vi "写入数据.vi"(8 "error in (no error)":errorcluster caption="错误输入（无错误）", 10 "数据":dbl[](array[numeric]), 11 "DAQ输入":refnum<class "DAQ.lvclass">) -> (0 "error out":errorcluster caption="错误输出", 3 "DAQ输出":refnum<class "DAQ.lvclass">)   [LabVIEW 2015]
uses:
  DAQ.lvclass
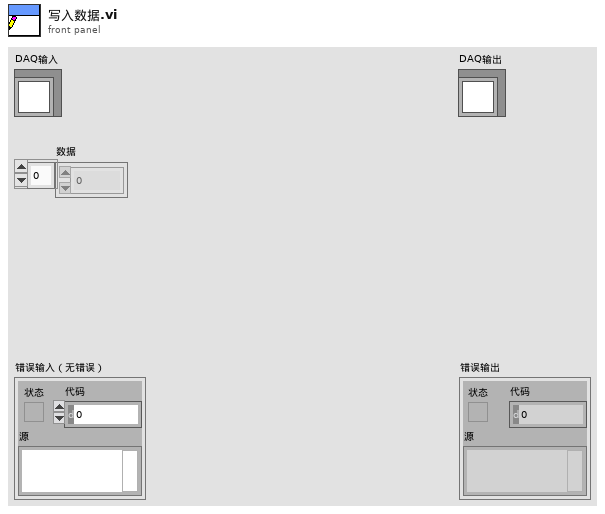
[diagram p1: front panel]
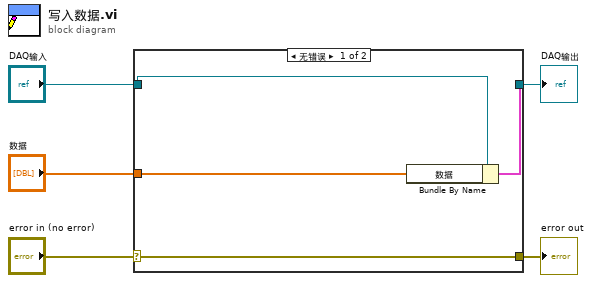
[diagram p0: block diagram]
diagram:
  n1 = case shown="无错误" "error in (no error)" {
    selector: "error in (no error)" -> [w9 w10]
    tunnel: [w9 w10] -> w4
    tunnel: [w7 w11] -> w2
    tunnel: "DAQ输入" -> [w8 w11]
    tunnel: "数据" -> [w6 _]
    frame No Error {
      n2 = Bundle By Name(cluster=w8, "数据"=w6) -> (w7:cluster{})
    }
    frame Error {
    }
  }
  "error out" <- w4
  "DAQ输出" <- w2
